vi "FormProductsTable.vi"() -> ()   [LabVIEW 2013]
uses:
  <vilib>/Utility/config.llb/NI_LVConfig.lvlib
panel:
  in  "选项卡控件":enum32{"操作步骤", "产品管理"}(tab)
  in  "第二段":T1
  in  "参数设定":string[][](table)
  in  "删除":bool
  in  "确定":bool
  in  "添加":bool
  in  "退出":bool
  in  "更新":bool
  in  "产品型号":string(combo)
  in  "操作步骤":T2
  in  "请输入添加的产品名称":string
  in  "请选择要删除的产品":string(combo)
  # "出厂检验台"
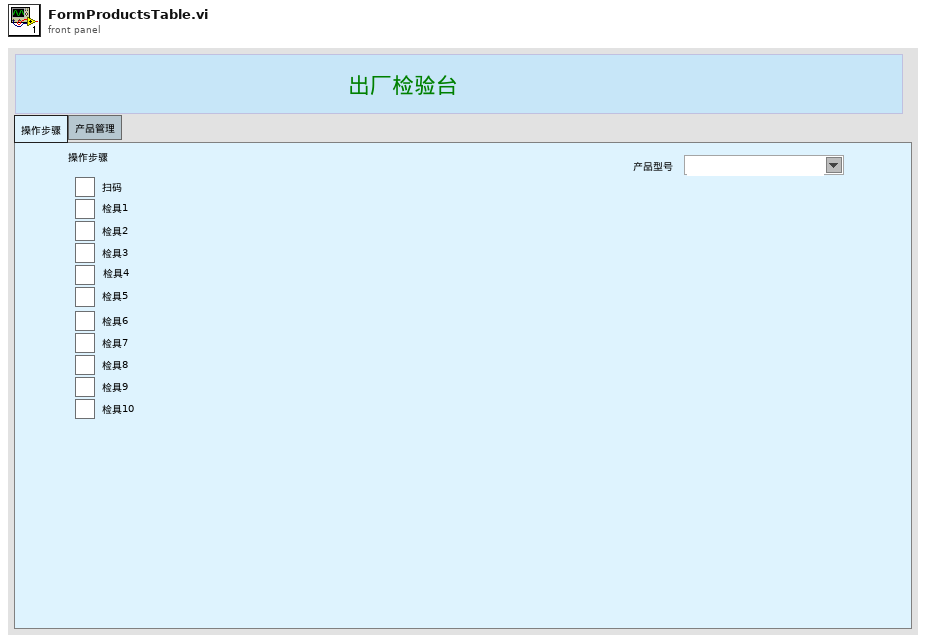
[diagram p1: front panel]
types:
  T1 = cluster{"检具6":bool, "检具7":bool, "检具8":bool, "检具9":bool, "检具10":bool}
  T2 = cluster{"扫码":bool, "检具1":bool, "检具2":bool, "检具3":bool, bool, "检具5":bool}
  T3 = typedef "NI_LVConfig.lvlib/Config Data RefNum.ctl" = refnum<k1>
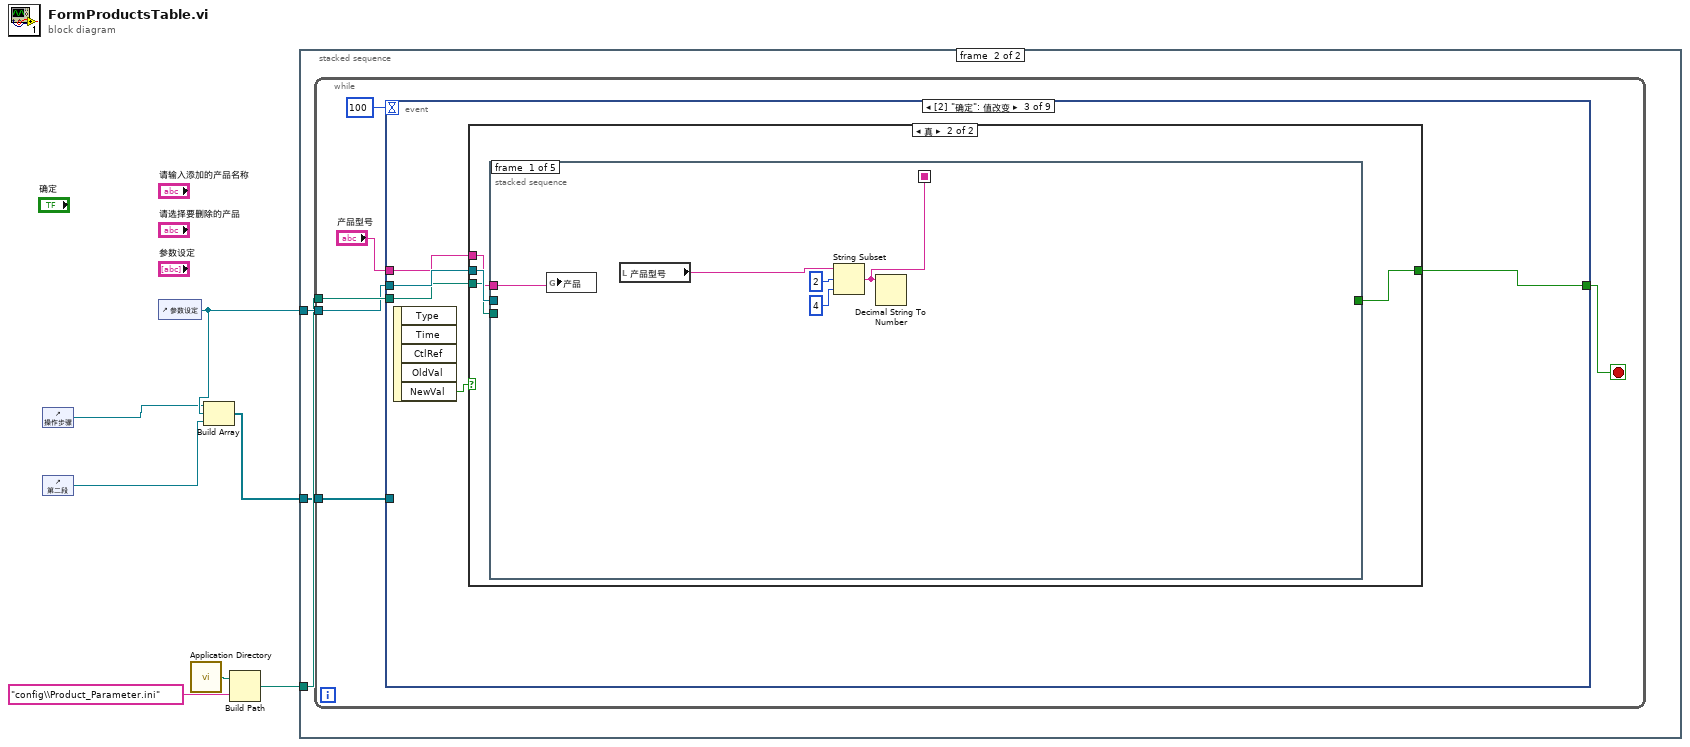
[diagram p0: block diagram]
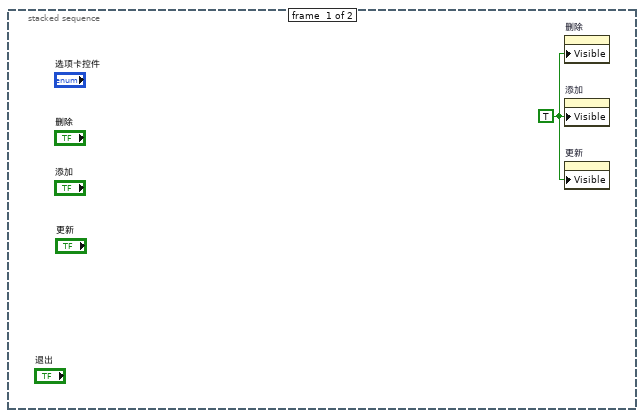
[diagram p2: hidden frame]
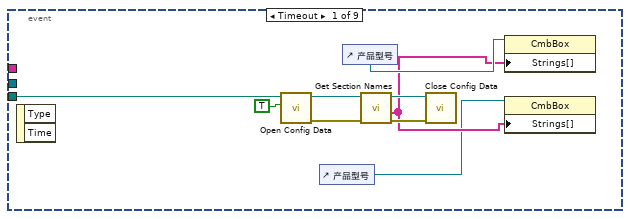
[diagram p3: hidden frame]
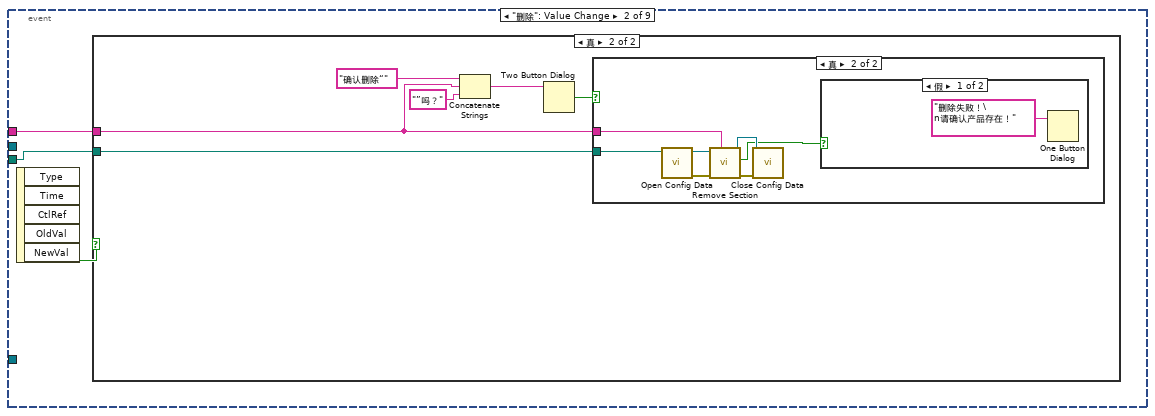
[diagram p4: hidden frame]
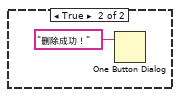
[diagram p7: hidden frame]
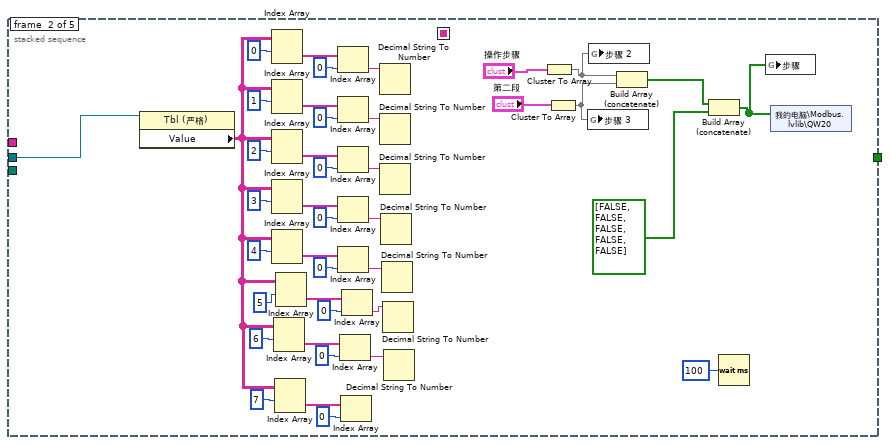
[diagram p9: hidden frame]
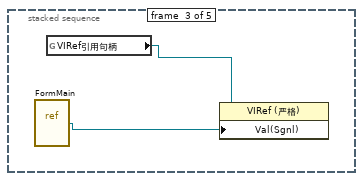
[diagram p10: hidden frame]
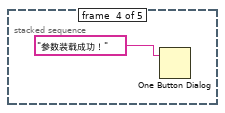
[diagram p11: hidden frame]
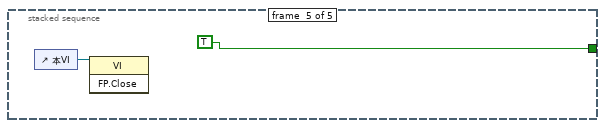
[diagram p12: hidden frame]
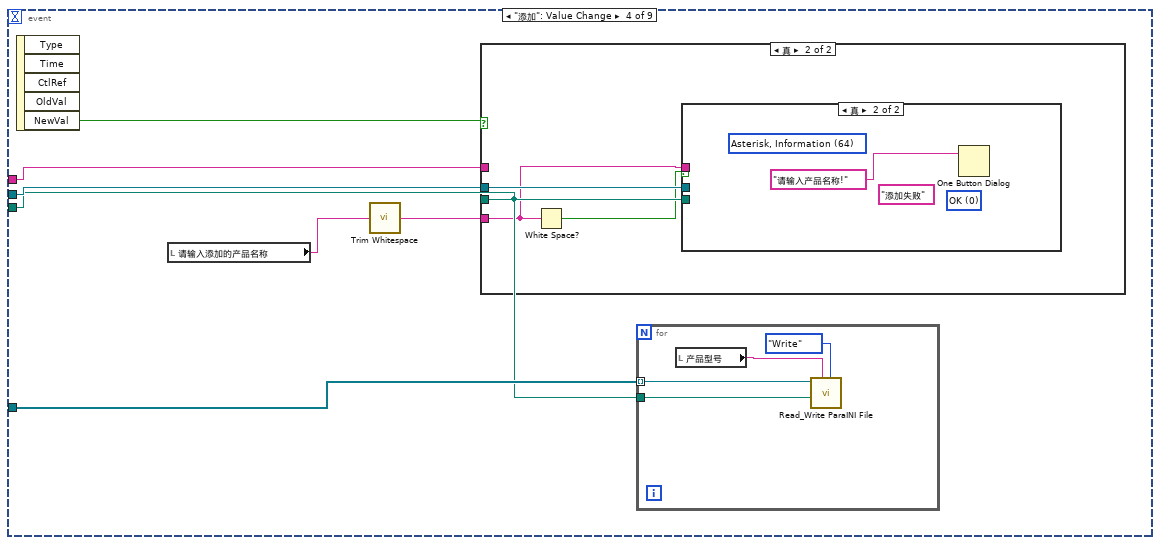
[diagram p13: hidden frame]
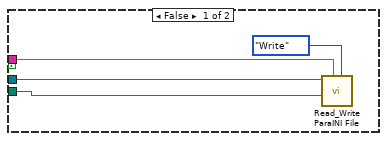
[diagram p15: hidden frame]
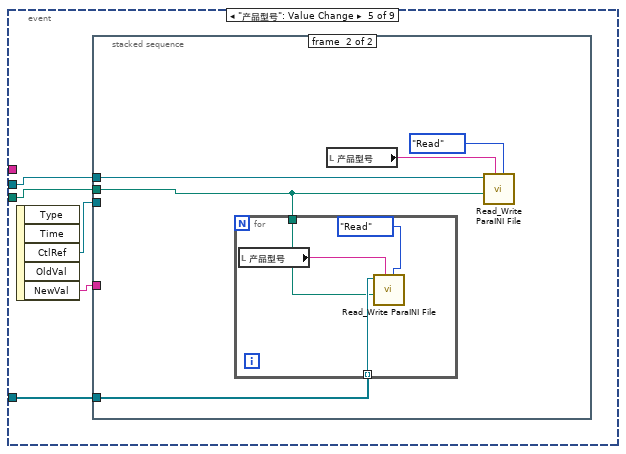
[diagram p16: hidden frame]
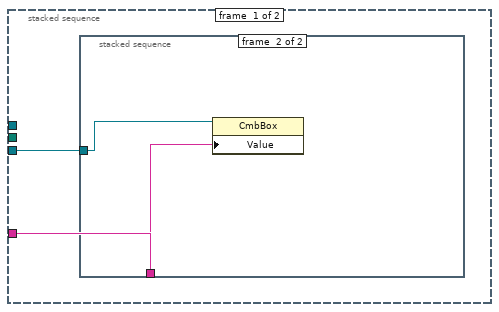
[diagram p17: hidden frame]
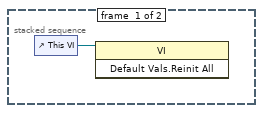
[diagram p18: hidden frame]
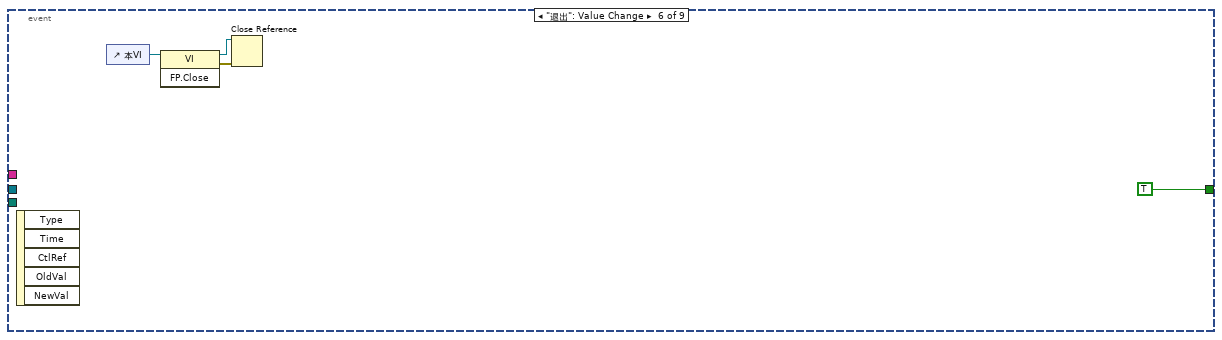
[diagram p19: hidden frame]
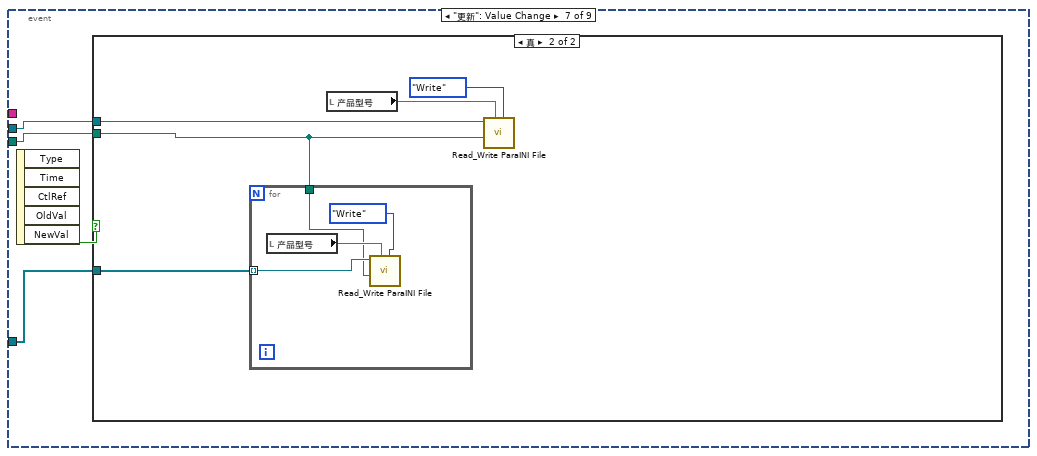
[diagram p20: hidden frame]
diagram:
  n1 = control-ref of="操作步骤"() -> (w5:refnum<vi>)
  n2 = control-ref of="第二段"() -> (w1:refnum<vi>)
  n3 = control-ref of="参数设定"() -> (w7:refnum<vi>)
  n4 = call <vilib>:"Application Directory.vi"() -> ("Application Directory"=w2:path)
  n5 = Build Array(w5, w7, w1) -> (w6:refnum<vi>[])
  n6 = Build Path(base path=w2, name or relative path="config\\Product_Parameter.ini" ("名称或相对路径")) -> (appended path=w4:path)
  n7 = stacked-sequence {
    tunnel: w7 -> [_ w11]
    tunnel: w4 -> [_ w10]
    tunnel: w6 -> [_ w9]
    frame #0 {
      w8 = TRUE ("可见")
      n8 = property on="删除" class="Bool (严格)"("Visible"=w8) -> ()  [unwired: 2 in, 2 out]
      n9 = property on="添加" class="Bool (严格)"("Visible"=w8) -> ()  [unwired: 2 in, 2 out]
      n10 = property on="更新" class="Bool (严格)"("Visible"=w8) -> ()  [unwired: 2 in, 2 out]
    }
    frame #1 {
      n11 = while {
        tunnel: w10 -> [w17]
        tunnel: w11 -> [w15]
        tunnel: w9 -> [w12]
        stop <- w16 stop-if-true
        n12 = event shown="[2] \"确定\": 值改变" {
          selector: _ -> [_ _ _ _ _ _ _ _ _]
          dyn-events: _ -> [_ _ _ _ _ _ _ _ _]
          timeout: 100 -> [_ _ _ _ _ _ _ _ _]
          tunnel: w17 -> [w21 w29 w46 w108 w128 _ w151 _ _]
          tunnel: [_ _ w48 _ _ TRUE _ _ TRUE] -> w16
          tunnel: w15 -> [_ _ w47 w111 w129 _ w150 _ _]
          tunnel: "产品型号" -> [_ w27 w45 w110 _ _ _ _ _]
          tunnel: w12 -> [_ _ _ w109 w125 _ w148 _ _]
          event Timeout {
            n13 = event-data() -> ()  [unwired: 1 in, 2 out]
            n14 = call <vilib>:"Open Config Data.vi"("create file if necessary (T)"=TRUE, "configuration file path"=w21) -> ("error out"=w23:errorcluster, "refnum"=w22:T3)  [unwired: 7 in, 1 out]
            n15 = control-ref of="产品型号"() -> (w18:refnum<vi>)
            n16 = control-ref of="产品型号"() -> (w20:refnum<vi>)
            n17 = call <vilib>:"Get Section Names.vi"("error in (no error)"=w23, "refnum"=w22) -> ("error out"=w25:errorcluster, "section names"=w19:string[], "refnum out"=w24:T3)  [unwired: 7 in]
            n18 = call <vilib>:"Close Config Data.vi"("error in (no error)"=w25, "refnum"=w24) -> ()  [unwired: 8 in, 2 out]
            n19 = property on="属性节点" class="CmbBox"(reference=w20, "Strings[]"=w19) -> ()  [unwired: 1 in, 2 out]
            n20 = property on="属性节点" class="CmbBox"(reference=w18, "Strings[]"=w19) -> ()  [unwired: 1 in, 2 out]
          }
          event "删除": Value Change {
            n21 = event-data() -> ("NewVal"=w28:bool)  [unwired: 1 in, 4 out]
            n22 = case shown="真" w28 {
              tunnel: w29 -> [_ w31]
              tunnel: w27 -> [_ w30]
              frame False {
              }
              frame True {
                n23 = Concatenate Strings("确认删除“", w30, "”吗？") -> (w33:string)
                n24 = Two Button Dialog(message=w33) -> (T button?=w32:bool)  [unwired: 2 in]
                n25 = case shown="真" w32 {
                  tunnel: w31 -> [_ w37]
                  tunnel: w30 -> [_ w36]
                  frame False {
                  }
                  frame True {
                    n26 = call <vilib>:"Open Config Data.vi"("configuration file path"=w37) -> ("error out"=w39:errorcluster, "refnum"=w42:T3)  [unwired: 8 in, 1 out]
                    n27 = call <vilib>:"Remove Section.vi"("section"=w36, "error in (no error)"=w39, "refnum"=w42) -> ("error out"=w41:errorcluster, "section exists?"=w38:bool, "refnum out"=w40:T3)  [unwired: 6 in]
                    n28 = call <vilib>:"Close Config Data.vi"("error in (no error)"=w41, "refnum"=w40) -> ()  [unwired: 8 in, 2 out]
                    n29 = case shown="假" w38 {
                      frame False {
                        n30 = One Button Dialog(message="删除失败！\n请确认产品存在！" ("消息")) -> ()  [unwired: 1 in, 1 out]
                      }
                      frame True {
                        n31 = One Button Dialog(message="删除成功！" ("消息")) -> ()  [unwired: 1 in, 1 out]
                      }
                    }
                  }
                }
              }
            }
          }
          event "确定": Value Change {
            n32 = event-data() -> ("NewVal"=w49:bool)  [unwired: 1 in, 4 out]
            n33 = case shown="真" w49 {
              tunnel: [_ w53] -> w48
              tunnel: w47 -> [_ w52]
              tunnel: w46 -> [_ w51]
              tunnel: w45 -> [_ w50]
              frame False {
              }
              frame True {
                n34 = stacked-sequence {
                  seq-local: [w58 _ _ _ _] -> [_ _ _ _ _]
                  tunnel: [_ _ _ _ TRUE] -> w53
                  tunnel: w52 -> [_ w65 _ _ _]
                  tunnel: w51 -> [_ _ _ _ _]
                  tunnel: w50 -> [w54 _ _ _ _]
                  frame #0 {
                    n35 = global write "全局 3.vi" "产品"(w54) -> ()
                    n36 = local read "产品型号"() -> (w57:string)
                    n37 = String Subset(string=w57, offset (0)=u16 2 ("偏移量(0)"), length (rest)=u16 4 ("长度（剩余）")) -> (substring=w58:string)
                    n38 = Decimal String To Number(string=w58) -> ()  [unwired: 2 in, 2 out]
                  }
                  frame #1 {
                    n39 = property class="Tbl (严格)"(reference=w65) -> ("Value"=w67:string[][])  [unwired: 1 in, 2 out]
                    n40 = Index Array(array=w67, index (row)=0 ("索引 (行)")) -> (element=w97:string[])  [unwired: 1 in]
                    n41 = Index Array(array=w67, index (row)=1 ("索引 (行)")) -> (element=w86:string[])  [unwired: 1 in]
                    n42 = Index Array(array=w67, index (row)=2 ("索引 (行)")) -> (element=w85:string[])  [unwired: 1 in]
                    n43 = Index Array(array=w67, index (row)=3 ("索引 (行)")) -> (element=w81:string[])  [unwired: 1 in]
                    n44 = Index Array(array=w67, index (row)=4 ("索引 (行)")) -> (element=w82:string[])  [unwired: 1 in]
                    n45 = Index Array(array=w67, index (row)=6 ("索引 (行)")) -> (element=w77:string[])  [unwired: 1 in]
                    n46 = Index Array(array=w67, index (row)=7 ("索引 (行)")) -> (element=w68:string[])  [unwired: 1 in]
                    n47 = Index Array(array=w67, index (row)=5 ("禁用的索引 (列)")) -> (element=w74:string[])  [unwired: 1 in]
                    n48 = Index Array(array=w97, index=0 ("索引")) -> (element=w98:string)
                    n49 = Index Array(array=w86, index=0 ("索引")) -> (element=w89:string)
                    n50 = Index Array(array=w85, index=0 ("索引")) -> (element=w88:string)
                    n51 = Index Array(array=w81, index=0 ("索引")) -> (element=w80:string)
                    n52 = Index Array(array=w82, index=0 ("索引")) -> (element=w79:string)
                    n53 = Index Array(array=w77, index=0 ("索引")) -> (element=w78:string)
                    n54 = Index Array(array=w68, index=0 ("索引")) -> ()  [unwired: 1 out]
                    n55 = Index Array(array=w74, index=0 ("索引")) -> (element=w72:string)
                    n56 = Decimal String To Number(string=w98) -> ()  [unwired: 2 in, 2 out]
                    n57 = Decimal String To Number(string=w89) -> ()  [unwired: 2 in, 2 out]
                    n58 = Decimal String To Number(string=w88) -> ()  [unwired: 2 in, 2 out]
                    n59 = Decimal String To Number(string=w80) -> ()  [unwired: 2 in, 2 out]
                    n60 = Decimal String To Number(string=w79) -> ()  [unwired: 2 in, 2 out]
                    n61 = Decimal String To Number(string=w72) -> ()  [unwired: 2 in, 2 out]
                    n62 = Decimal String To Number(string=w78) -> ()  [unwired: 2 in, 2 out]
                    n63 = Cluster To Array(cluster="操作步骤") -> (array=w60:bool[])
                    n64 = Cluster To Array(cluster="第二段") -> (array=w59:bool[])
                    n65 = global write "全局 3.vi" "步骤 3"(w59) -> ()
                    n66 = global write "全局 3.vi" "步骤 2"(w60) -> ()
                    n67 = Build Array (concatenate)(w60, w59) -> (w62:bool[])
                    n68 = Build Array (concatenate)(w62, bool[] [FALSE, FALSE, FALSE, FALSE, FALSE] ("数组")) -> (w61:bool[])
                    n69 = Wait (ms)(milliseconds to wait=u32 100) -> ()  [unwired: 1 out]
                    n70 = global write "全局 3.vi" "步骤"(w61) -> ()
                    n71 = shared-variable "我的电脑\\Modbus.lvlib\\QW20"(w61) -> ()  [unwired: 1 in, 1 out]
                  }
                  frame #2 {
                    n72 = vi-ref "FormMain.vi"() -> (w101:refnum<vi>)
                    n73 = global read "全局 3.vi" "VIRef引用句柄"() -> (w100:refnum<vi>)
                    n74 = property class="VIRef (严格)"(reference=w100, "Val(Sgnl)"=w101) -> ()  [unwired: 1 in, 2 out]
                  }
                  frame #3 {
                    n75 = One Button Dialog(message="参数装载成功！" ("消息")) -> ()  [unwired: 1 in, 1 out]
                  }
                  frame #4 {
                    n76 = control-ref of="本VI"() -> (w103:refnum<vi>)
                    n77 = invoke class="VI" method="FP.Close"(reference=w103) -> ()  [unwired: 2 in, 3 out]
                  }
                }
              }
            }
          }
          event "添加": Value Change {
            n78 = event-data() -> ("NewVal"=w107:bool)  [unwired: 1 in, 4 out]
            n79 = local read "请输入添加的产品名称"() -> (w106:string)
            n80 = call <vilib>:"Trim Whitespace.vi"("string"=w106) -> ("trimmed string"=w105:string)  [unwired: 1 in]
            n81 = case shown="真" w107 {
              tunnel: w111 -> [_ w119]
              tunnel: w108 -> [_ w118]
              tunnel: w110 -> [_ _]
              tunnel: w105 -> [_ w116]
              frame False {
              }
              frame True {
                n82 = White Space?(1:w116) -> (0:w117:bool)
                n83 = case shown="真" w117 {
                  tunnel: w119 -> [w123 _]
                  tunnel: w118 -> [w122 _]
                  tunnel: w116 -> [w121 _]
                  frame False {
                    n84 = call "Read_Write ParaINI File.vi"("Mode"=enum16{"Read", "Write"}."Write", "Section"=w121, "Filepath"=w122, "Ctl Refnum"=w123) -> ()  [unwired: 7 in, 1 out]
                  }
                  frame True {
                    (unwired) 64 items=["None"=0, "Hand, Error, Stop"=16, "Question"=32, "Exclamation, Warning"=48, "Asterisk, Information"=64] ("icon")
                    (unwired) 0 items=["OK", "OKCancel", "AbortRetryIgnore", "YesNoCancel", "YesNo", "RetryCancel"] ("buttons")
                    (unwired) "添加失败" ("caption")
                    n85 = One Button Dialog(message="请输入产品名称!" ("text")) -> ()  [unwired: 1 in, 1 out]
                  }
                }
              }
            }
            n86 = for {
              tunnel: w109 -> [w113] mode=indexing
              tunnel: w108 -> [w112]
              n87 = local read "产品型号"() -> (w114:string)
              n88 = call "Read_Write ParaINI File.vi"("Mode"=enum16{"Read", "Write"}."Write", "Section"=w114, "Filepath"=w112, "Ctl Refnum"=w113) -> ()  [unwired: 7 in, 1 out]
            }
          }
          event "产品型号": Value Change {
            n89 = event-data() -> ("CtlRef"=w127:refnum<vi>, "NewVal"=w126:string)  [unwired: 1 in, 3 out]
            n90 = stacked-sequence {
              tunnel: w129 -> [_ w139]
              tunnel: w128 -> [_ w135]
              tunnel: w127 -> [w131 _]
              tunnel: w126 -> [w130 _]
              tunnel: w125 -> [_ w136]
              frame #0 {
                n91 = stacked-sequence {
                  tunnel: w131 -> [_ w133]
                  tunnel: w130 -> [_ w134]
                  frame #0 {
                    n92 = control-ref of="This VI"() -> (w132:refnum<vi>)
                    n93 = invoke class="VI" method="Default Vals.Reinit All"(reference=w132) -> ()  [unwired: 2 in, 3 out]
                  }
                  frame #1 {
                    n94 = property class="CmbBox"(reference=w133, "Value"=w134) -> ()  [unwired: 1 in, 2 out]
                  }
                }
              }
              frame #1 {
                n95 = for {
                  tunnel: w136 -> [w142] mode=indexing
                  tunnel: w135 -> [w141]
                  n96 = local read "产品型号"() -> (w140:string)
                  n97 = call "Read_Write ParaINI File.vi"("Mode"=enum16{"Read", "Write"}."Read", "Section"=w140, "Filepath"=w141, "Ctl Refnum"=w142) -> ()  [unwired: 7 in, 1 out]
                }
                n98 = local read "产品型号"() -> (w137:string)
                n99 = call "Read_Write ParaINI File.vi"("Mode"=enum16{"Read", "Write"}."Read", "Section"=w137, "Filepath"=w135, "Ctl Refnum"=w139) -> ()  [unwired: 7 in, 1 out]
              }
            }
          }
          event "退出": Value Change {
            n100 = event-data() -> ()  [unwired: 1 in, 5 out]
            n101 = control-ref of="本VI"() -> (w146:refnum<vi>)
            n102 = invoke class="VI" method="FP.Close"(reference=w146) -> (reference out=w144:refnum<vi>, error out=w145:errorcluster)  [unwired: 2 in, 1 out]
            n103 = Close Reference(reference=w144, error in (no error)=w145) -> ()  [unwired: 1 out]
          }
          event "更新": Value Change {
            n104 = event-data() -> ("NewVal"=w149:bool)  [unwired: 1 in, 4 out]
            n105 = case shown="真" w149 {
              tunnel: w151 -> [_ w152]
              tunnel: w150 -> [_ w156]
              tunnel: w148 -> [_ w153]
              frame False {
              }
              frame True {
                n106 = for {
                  tunnel: w153 -> [w158] mode=indexing
                  tunnel: w152 -> [w157]
                  n107 = local read "产品型号"() -> (w159:string)
                  n108 = call "Read_Write ParaINI File.vi"("Mode"=enum16{"Read", "Write"}."Write", "Section"=w159, "Filepath"=w157, "Ctl Refnum"=w158) -> ()  [unwired: 7 in, 1 out]
                }
                n109 = local read "产品型号"() -> (w155:string)
                n110 = call "Read_Write ParaINI File.vi"("Mode"=enum16{"Read", "Write"}."Write", "Section"=w155, "Filepath"=w152, "Ctl Refnum"=w156) -> ()  [unwired: 7 in, 1 out]
              }
            }
          }
          event "请输入添加的产品名称": Value Change {
            n111 = event-data() -> ("OldVal"=w163:string)  [unwired: 1 in, 5 out]
            n112 = control-ref of="产品型号"() -> (w161:refnum<vi>)
            n113 = property on="属性节点" class="CmbBox"(reference=w161) -> ("Strings[]"=w162:string[])  [unwired: 1 in, 2 out]
            n114 = for {
              tunnel: w163 -> [w164]
              tunnel: w162 -> [w165] mode=indexing
              n115 = Equal?(x=w164, y=w165) -> (x = y?=w166:bool)
              n116 = case shown="真" w166 {
                tunnel: w164 -> [_ w167]
                frame False {
                }
                frame True {
                  n117 = stacked-sequence {
                    tunnel: w167 -> [w170 _]
                    frame #0 {
                      (unwired) 64 items=["None"=0, "Hand, Error, Stop"=16, "Question"=32, "Exclamation, Warning"=48, "Asterisk, Information"=64] ("icon")
                      n118 = Concatenate Strings("已经存在产品”" ("text"), w170, "“\n请勿重复添加！" ("字符串")) -> (w168:string)
                      n119 = One Button Dialog(message=w168) -> ()  [unwired: 1 in, 1 out]
                    }
                    frame #1 {
                      n120 = local write "请输入添加的产品名称"("" ("请输入添加的产品名称")) -> ()
                    }
                  }
                }
              }
            }
          }
          event Panel Close {
            n121 = event-data() -> ()  [unwired: 1 in, 3 out]
          }
        }
      }
    }
  }
